vi "Arrange Terminals.vi"(8 "error in (no error)":errorcluster, 10 "Horizontal Only? (F)":bool, 11 "Diagram in":refnum<vi>) -> (0 "error out":errorcluster, 3 "Diagram out":refnum<vi>)   [LabVIEW 2019, in "Builtins.lvlib"]
doc: "Aligns the selected front panel or block diagram objects excluding any display objects (i.e. labels, captions, inc/dec buttons, etc.)\n\nCreated by: Ryan Pacini"
uses:
  Builtins.lvlib
  Arrange.ctl
  Label Position.ctl
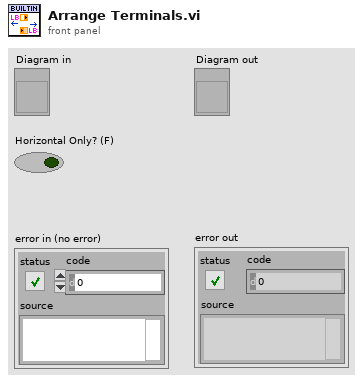
[diagram p1: front panel]
types:
  T1 = typedef "Builtins.lvlib/Arrange.ctl" = enum8{"left_to_right", "right_to_left"}
  T2 = typedef "Builtins.lvlib/Label Position.ctl" = enum8{"Unchanged", "Top-left", "Top-middle", "Top-right", "Right-top", "Right-middle", "Right-bottom", "Bottom-right", "Bottom-middle", "Bottom-left", "Left-bottom", "Left-middle", "Left-top"}
  T3 = typedef "LVRectTypeDef.ctl" = cluster{"Left":i16, "Top":i16, "Right":i16, "Bottom":i16}
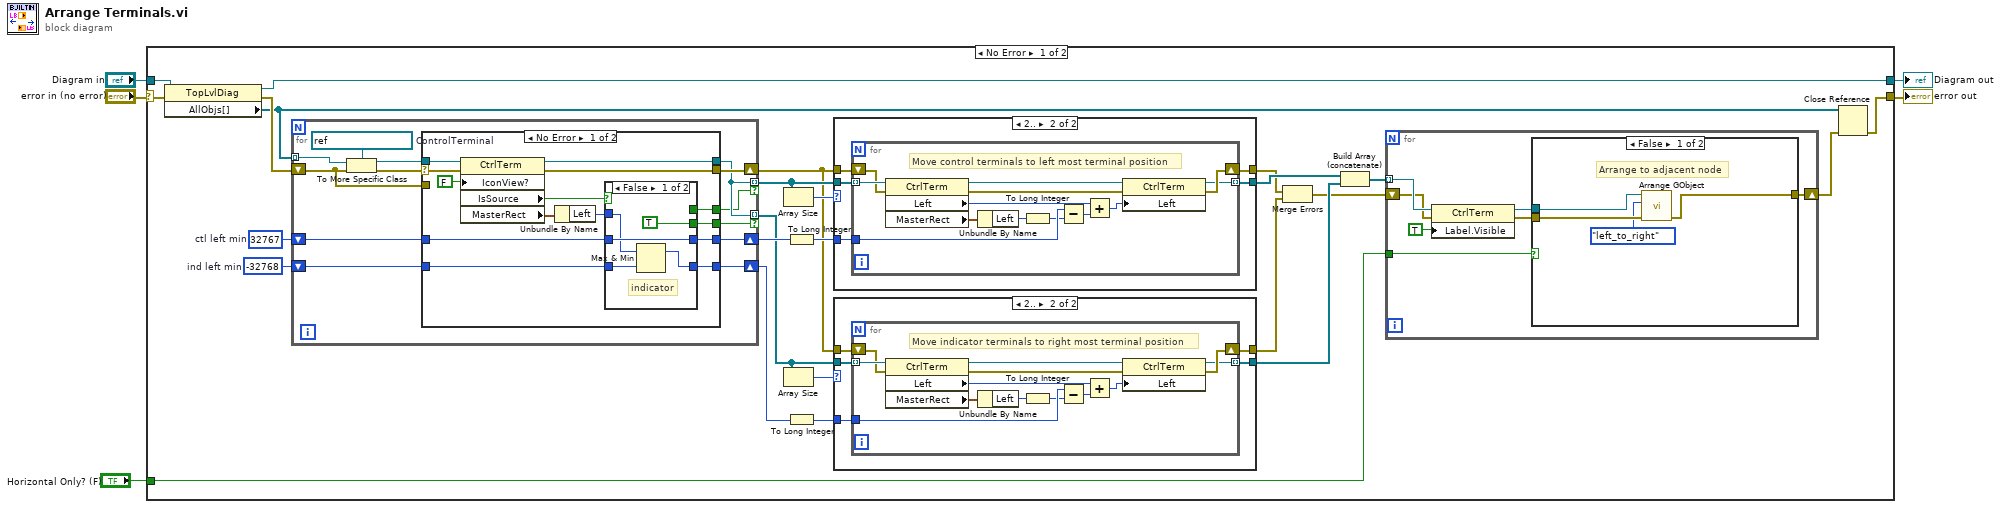
[diagram p0: block diagram]
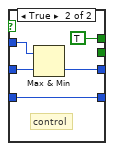
[diagram p3: hidden frame]
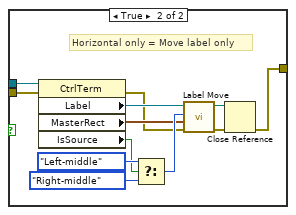
[diagram p6: hidden frame]
diagram:
  n1 = case shown="No Error" "error in (no error)" {
    selector: "error in (no error)" -> [w11 w134]
    tunnel: "Diagram in" -> [w12 w135]
    tunnel: [w6 w135] -> w4
    tunnel: [w29 w134] -> w3
    tunnel: "Horizontal Only? (F)" -> [w10 _]
    frame No Error {
      w23 = i16 -32768  # ind left min
      w24 = i16 32767  # ctl left min
      n2 = property class="TopLvlDiag"(reference=w12, error in=w11) -> (reference out=w6:refnum<vi>, error out=w28:errorcluster, "AllObjs[]"=w7:refnum<vi>[])
      n3 = for {
        tunnel: w7 -> [w63] mode=indexing
        shift-right: [w58] -> w20
        shift-left: w28 -> [w59]
        tunnel: [w57] -> w27 mode=indexing if=w54
        tunnel: [w57] -> w18 mode=indexing if=w51
        shift-right: [w56] -> w22
        shift-left: w24 -> [w55]
        shift-right: [w52] -> w16
        shift-left: w23 -> [w53]
        w62 = refnum<vi> refnum  # ControlTerminal
        n4 = To More Specific Class(target class=w62, reference=w63, error in=w59) -> (specific class reference=w61:refnum<vi>, error out=w60:errorcluster)
        n5 = case shown="No Error" w60 {
          selector: w60 -> [w76 _]
          tunnel: w61 -> [w77 _]
          tunnel: w59 -> [_ w90]
          tunnel: [w74 w90] -> w58
          tunnel: [w75 _] -> w57
          tunnel: [w69 w89] -> w56
          tunnel: w55 -> [w68 w89]
          tunnel: [w67 _] -> w54
          tunnel: w53 -> [w66 w88]
          tunnel: [w65 w88] -> w52
          tunnel: [w64 _] -> w51
          frame No Error {
            n6 = property class="CtrlTerm"(reference=w77, error in=w76, "IconView?"=FALSE ("Icon View?")) -> (reference out=w75:refnum<vi>, error out=w74:errorcluster, "IsSource"=w72:bool, "MasterRect"=w71:T3)
            n7 = Unbundle By Name(w71) -> ("Left"=w70:i16)
            n8 = case shown="False" w72 {
              tunnel: w70 -> [w80 w87]
              tunnel: [w82 w86] -> w69
              tunnel: w68 -> [w82 w85]
              tunnel: [_ TRUE] -> w67
              tunnel: w66 -> [w81 w83]
              tunnel: [w78 w83] -> w65
              tunnel: [TRUE _] -> w64
              frame False {
                # "indicator"
                n9 = Max & Min(x=w80, y=w81) -> (max(x,y)=w78:i16)  [unwired: 1 out]
              }
              frame True {
                # "control"
                n10 = Max & Min(x=w87, y=w85) -> (min(x,y)=w86:i16)  [unwired: 1 out]
              }
            }
          }
          frame Error {
          }
        }
      }
      n11 = Array Size(array=w27) -> (size(s)=w26:i32)
      n12 = Array Size(array=w18) -> (size(s)=w19:i32)
      n13 = To Long Integer(number=w22) -> (32bit integer=w21:i32)
      n14 = To Long Integer(number=w16) -> (32bit integer=w17:i32)
      n15 = case shown="2.." w26 {
        tunnel: w21 -> [_ w97]
        tunnel: w27 -> [w91 w96]
        tunnel: w20 -> [w92 w95]
        tunnel: [w92 w94] -> w15
        tunnel: [w91 w93] -> w25
        frame ..1 {
        }
        frame 2.. {
          n16 = for {
            tunnel: w96 -> [w110] mode=indexing
            tunnel: w97 -> [w101]
            shift-right: [w109] -> w94
            shift-left: w95 -> [w106]
            tunnel: [w108] -> w93 mode=indexing
            # "Move control terminals to left most terminal position"
            n17 = property class="CtrlTerm"(reference=w110, error in=w106) -> (reference out=w107:refnum<vi>, error out=w103:errorcluster, "Left"=w104:i32, "MasterRect"=w102:T3)
            n18 = Unbundle By Name(w102) -> ("Left"=w100:i16)
            n19 = To Long Integer(number=w100) -> (32bit integer=w98:i32)
            n20 = Subtract(x=w101, y=w98) -> (x-y=w99:i32)
            n21 = Add(x=w104, y=w99) -> (x+y=w105:i32)
            n22 = property class="CtrlTerm"(reference=w107, error in=w103, "Left"=w105) -> (reference out=w108:refnum<vi>, error out=w109:errorcluster)
          }
        }
      }
      n23 = case shown="2.." w19 {
        tunnel: w17 -> [_ w37]
        tunnel: w18 -> [w31 w36]
        tunnel: w20 -> [w32 w35]
        tunnel: [w32 w34] -> w14
        tunnel: [w31 w33] -> w13
        frame ..1 {
        }
        frame 2.. {
          n24 = for {
            tunnel: w36 -> [w50] mode=indexing
            tunnel: w37 -> [w41]
            shift-right: [w49] -> w34
            shift-left: w35 -> [w46]
            tunnel: [w48] -> w33 mode=indexing
            # "Move indicator terminals to right most terminal position"
            n25 = property class="CtrlTerm"(reference=w50, error in=w46) -> (reference out=w47:refnum<vi>, error out=w43:errorcluster, "Left"=w44:i32, "MasterRect"=w42:T3)
            n26 = Unbundle By Name(w42) -> ("Left"=w40:i16)
            n27 = To Long Integer(number=w40) -> (32bit integer=w38:i32)
            n28 = Subtract(x=w41, y=w38) -> (x-y=w39:i32)
            n29 = Add(x=w44, y=w39) -> (x+y=w45:i32)
            n30 = property class="CtrlTerm"(reference=w47, error in=w43, "Left"=w45) -> (reference out=w48:refnum<vi>, error out=w49:errorcluster)
          }
        }
      }
      n31 = Merge Errors(w15, w14) -> (w9:errorcluster)
      n32 = Build Array (concatenate)(w25, w13) -> (w8:refnum<vi>[])
      n33 = for {
        tunnel: w8 -> [w117] mode=indexing
        shift-right: [w112] -> w30
        shift-left: w9 -> [w116]
        tunnel: w10 -> [w111]
        n34 = property class="CtrlTerm"(reference=w117, error in=w116, "Label.Visible"=TRUE) -> (reference out=w113:refnum<vi>, error out=w114:errorcluster)
        n35 = case shown="False" w111 {
          tunnel: w114 -> [w121 w127]
          tunnel: w113 -> [w120 w126]
          tunnel: [w119 w129] -> w112
          frame False {
            # "Arrange to adjacent node"
            n36 = call "Arrange GObject.vi"("error in (no error)"=w121, "Arrange"=Arrange."left_to_right", "GObject in"=w120) -> ("error out"=w119:errorcluster)  [unwired: 6 in, 2 out]
          }
          frame True {
            # "Horizontal only = Move label only"
            n37 = property class="CtrlTerm"(reference=w126, error in=w127) -> (error out=w122:errorcluster, "Label"=w125:refnum<vi>, "MasterRect"=w124:T3, "IsSource"=w123:bool)  [unwired: 1 out]
            n38 = Select(t=Label_Position."Left-middle" ("Label Position"), s=w123, f=Label_Position."Right-middle" ("Label Position")) -> (s? t:f=w130:T2)
            n39 = call "Label Move.vi"("error in (no error)"=w122, "Owner Master Bounds Rect"=w124, "Label Position"=w130, "Label in"=w125) -> ("error out"=w133:errorcluster, "dup Label"=w128:refnum<vi>)  [unwired: 6 in]
            n40 = Close Reference(reference=w128, error in (no error)=w133) -> (error out=w129:errorcluster)
          }
        }
      }
      n41 = Close Reference(reference=w7, error in (no error)=w30) -> (error out=w29:errorcluster)
    }
    frame Error {
    }
  }
  "Diagram out" <- w4
  "error out" <- w3
